vi "ReadScopeFile.vi"(1 "本次文件名":string) -> ()   [LabVIEW 2018]
uses:
  Init/AllPath.vi
  <vilib>/Utility/file.llb/Read Delimited Spreadsheet (string).vi
  HistoryFile.vi
panel:
  out "波形图":waveform(dbl)(graph)
  out "数字":dbl[][](array[numeric])
  out "重复频率":string
  out "脉冲宽度":string
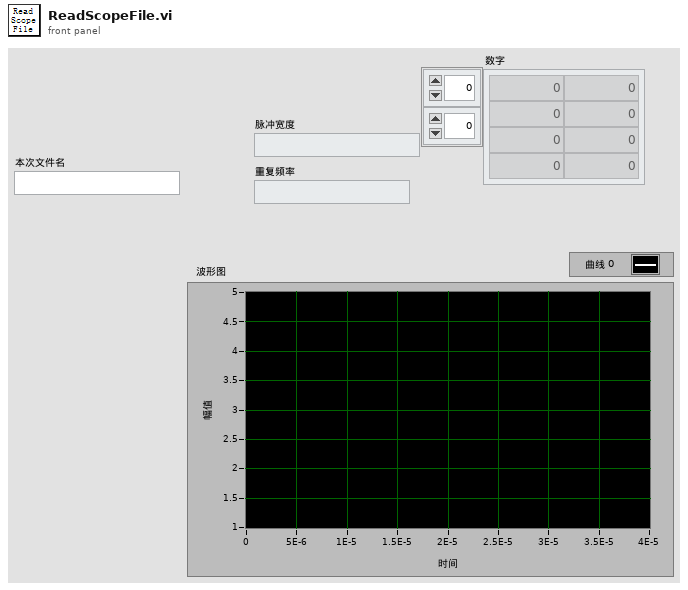
[diagram p1: front panel]
types:
  T1 = cluster{"能量/功率":path, " 示波器":path, " 光谱仪":path, "偏振":path, "近远场":cluster{" 近场图片":path, " 远场图片":path, "发散角数据":path}, "参数":path, " 基路径":path, "文件名信息":path, "输出模板路径":path, "输出报告路径":path}
  T2 = cluster{"波形":waveform(dbl), "脉宽":string, "重频":string, "脉冲宽度Uint":string, "重复频率Uint":string}
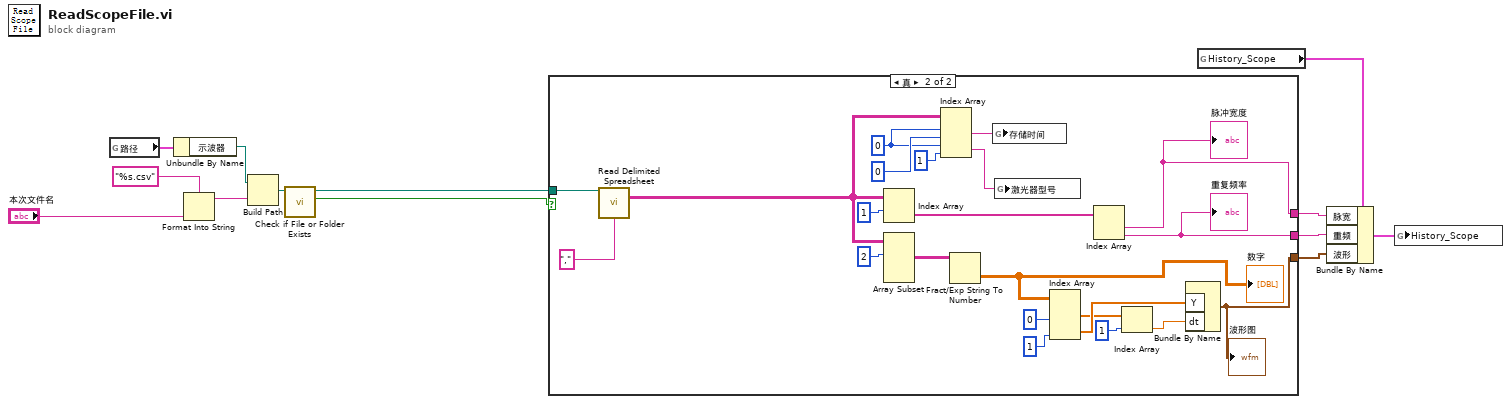
[diagram p0: block diagram]
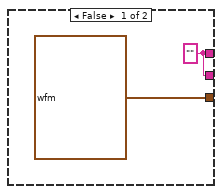
[diagram p2: hidden frame]
diagram:
  n1 = global read "AllPath.vi" "路径"() -> (w13:T1)
  n2 = Unbundle By Name(w13) -> ("示波器"=w12:path)
  n3 = Format Into String(format string="%s.csv" ("格式字符串"), "本次文件名") -> (resulting string=w9:string)  [unwired: 2 in, 1 out]
  n4 = Build Path(base path=w12, name or relative path=w9) -> (appended path=w3:path)
  n5 = call <vilib>:"Check if File or Folder Exists.vi"("path"=w3) -> ("file or folder exists?"=w1:bool, "dup path"=w2:path)  [unwired: 8 in, 1 out]
  n6 = case shown="真" w1 {
    tunnel: w2 -> [_ w37]
    tunnel: [w15 w24] -> w6
    tunnel: [w15 w23] -> w5
    tunnel: [waveform(dbl) {"t0"=timestamp(0 s since 1904-01-01), "dt"=1.0, "Y"=[]} w22] -> w4
    frame False {
      w15 = ""
    }
    frame True {
      w18 = 0 ("索引 (行)")
      n7 = call-poly <vilib>:"Read Delimited Spreadsheet.vi"("file path (dialog if empty)"=w37, "delimiter (\\t)"="," ("delimiter (\\t)")) -> ("all rows"=w21:string[][])  [unwired: 8 in, 5 out]
      n8 = Index Array(array=w21, index (row)=1 ("索引 (行)")) -> (element=w34:string[])  [unwired: 1 in]
      n9 = Array Subset(array=w21, index (row)=2 ("索引")) -> (w32:string[][])  [unwired: 3 in]
      n10 = Index Array(array=w21, index (row) #1=w18, index (col) #1=0 ("禁用的索引 (列)"), index (row) #2=w18, index (col) #2=1 ("禁用的索引 (列)")) -> (element #1=w19:string, element #2=w16:string)
      n11 = Fract/Exp String To Number(string=w32) -> (number=w31:dbl[][])  [unwired: 3 in, 1 out]
      "数字" <- w31
      n12 = global write "HistoryFile.vi" "存储时间"(w19) -> ()
      n13 = global write "HistoryFile.vi" "激光器型号"(w16) -> ()
      n14 = Index Array(array=w31, index (col) #1=0 ("禁用的索引 (列)"), index (col) #2=1 ("索引 (列)")) -> (element #1=w27:dbl[], element #2=w30:dbl[])  [unwired: 2 in]
      n15 = Index Array(array=w34) -> (element #1=w24:string, element #2=w23:string)  [unwired: 2 in]
      "脉冲宽度" <- w24
      "重复频率" <- w23
      n16 = Index Array(array=w27, index=1 ("索引")) -> (element=w25:dbl)
      n17 = Bundle By Name("Y"=w30, "dt"=w25) -> (w22:waveform(dbl))  [unwired: 1 in]
      "波形图" <- w22
    }
  }
  n18 = global read "HistoryFile.vi" "History_Scope"() -> (w8:T2)
  n19 = Bundle By Name(cluster=w8, "脉宽"=w6, "重频"=w5, "波形"=w4) -> (w7:T2)
  n20 = global write "HistoryFile.vi" "History_Scope"(w7) -> ()
